vi "Array Tests.vi"() -> ()   [LabVIEW 2020, in "CDM-Config.lvlib"]
uses:
  CDM-Config.lvlib
  Config-JSON/Config-JSON.lvclass
  Config Manager/Config Manager.lvclass
  Config Element/Config Element.lvclass
  <vilib>/JDP Science/JSONtext/JSONtext.lvlib
panel:
  out "Array":string[](array[string])
  out "JSON":string
  in  "Tree":string(tree)
  in  "String":string="{\n\"Beta\": {\"Foo\": \"Bar\"},\n\"Alpha\": [\"Alpha\", \"Beta\", \"Gamma\", \"Delta\"]\n}"
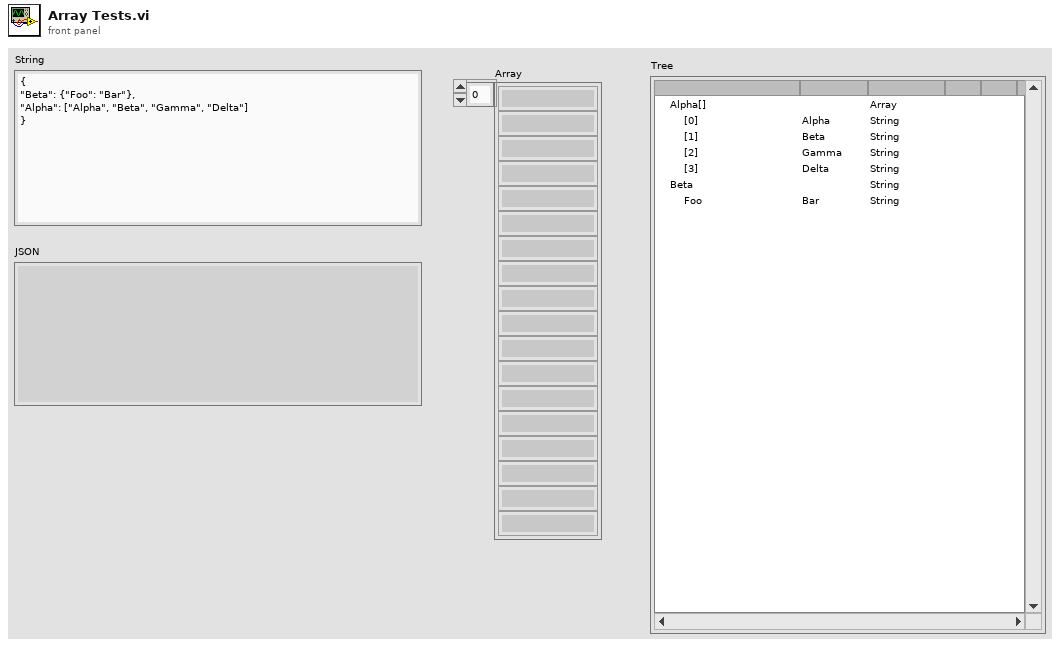
[diagram p1: front panel]
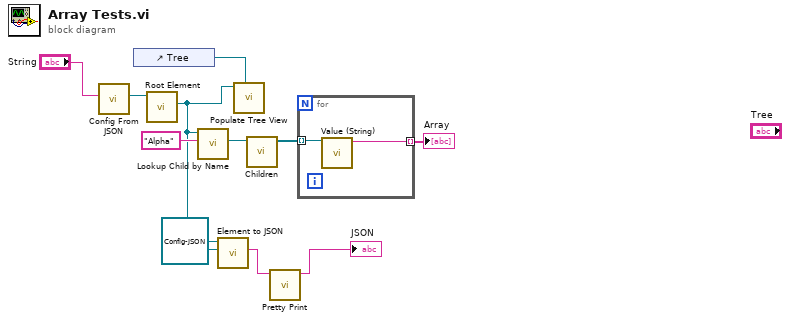
[diagram p0: block diagram]
diagram:
  n1 = call "Config From JSON.vi"("JSON"="String") -> ("Config"=w10:refnum<class "Config Manager.lvclass">)  [unwired: 9 in, 1 out]
  n2 = control-ref of="Tree"() -> (w6:refnum<vi>)
  n3 = call "Root Element.vi"("Config Manager in"=w10) -> ("Root Element"=w5:refnum<class "Config Element.lvclass">)  [unwired: 8 in, 2 out]
  n4 = call "Lookup Child by Name.vi"("Name"="Alpha", "Config Element in"=w5) -> ("Child"=w8:refnum<class "Config Element.lvclass">)  [unwired: 6 in, 3 out]
  n5 = call "Element to JSON.vi"("Element"=w5, "Config-JSON"=refnum<class "Config-JSON.lvclass"> refnum) -> ("JSON"=w3:string)  [unwired: 8 in, 1 out]
  n6 = call "Populate Tree View.vi"("Tree"=w6, "Element"=w5) -> ()  [unwired: 9 in, 1 out]
  n7 = call "Children.vi"("Config Element in"=w8) -> ("Elements"=w7:refnum<class "Config Element.lvclass">[])  [unwired: 9 in, 1 out]
  n8 = call <vilib>:"Pretty Print.vi"("JSON"=w3) -> ("<JSON>"=→"JSON":string)  [unwired: 8 in, 2 out]
  n9 = for {
    tunnel: w7 -> [w13] mode=indexing
    tunnel: [w12] -> w1 mode=indexing
    n10 = call "Value (String).vi"("Config Element in"=w13) -> ("String Value"=w12:string)  [unwired: 9 in, 1 out]
  }
  "Array" <- w1
